vi "PB_Nest_Loops.vi"(2 "error in (no error)":errorcluster, 3 "PB VLIW Array in":T1(array[cluster]) {"Output Bits" format="%x"}) -> (0 "error out":errorcluster, 1 "PB VLIW Array out":T1(array[cluster]) {"Output Bits" format="%x"})   [LabVIEW 2013, in "PulseBlaster.lvlib"]
uses:
  PulseBlaster.lvlib
  <vilib>/ErrorRing/Error Ring.xnode
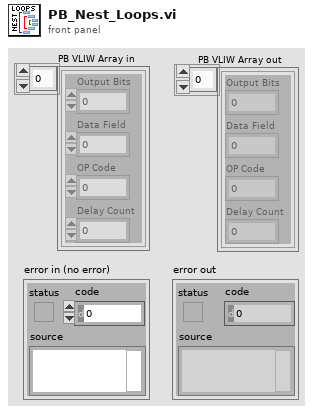
[diagram p1: front panel]
types:
  T1 = cluster{"Output Bits":u32, "Data Field":u32, "OP Code":u8, "Delay Count":u64}[]
  T2 = cluster{"Output Bits":u32, "Data Field":u32, "OP Code":u8, "Delay Count":u64}
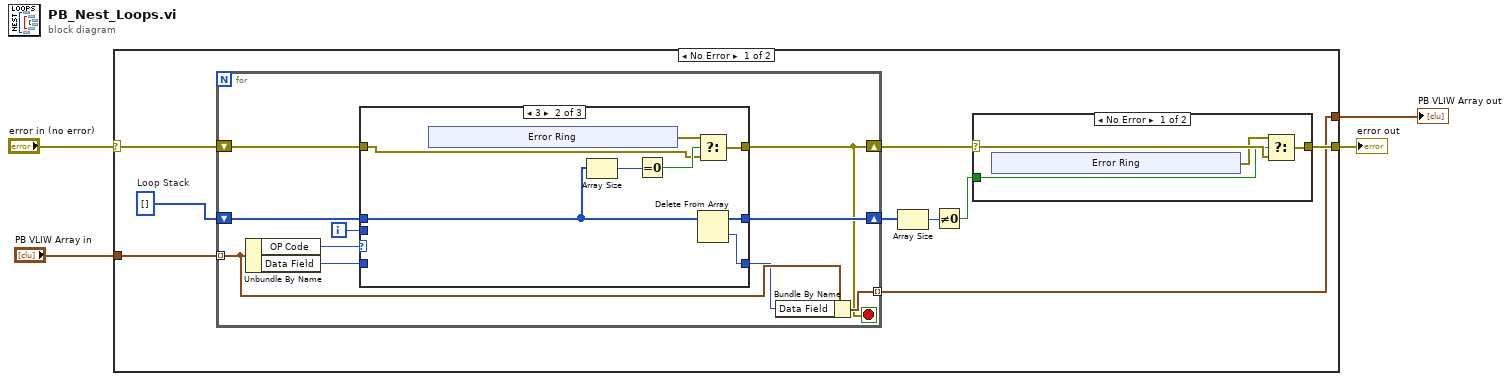
[diagram p0: block diagram]
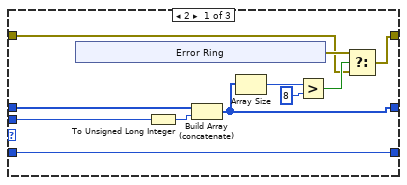
[diagram p3: hidden frame]
diagram:
  n1 = case shown="No Error" "error in (no error)" {
    selector: "error in (no error)" -> [w13 w55]
    tunnel: [w9 w55] -> w3
    tunnel: "PB VLIW Array in" -> [w12 w54]
    tunnel: [w5 w54] -> w1
    frame No Error {
      w11 = u32[] []  # Loop Stack
      n2 = for {
        shift-right: [w20] -> w10
        shift-left: w13 -> [w22]
        shift-right: [w23] -> w7
        shift-left: w11 -> [w24]
        tunnel: w12 -> [w28] mode=indexing
        tunnel: [w21] -> w5 mode=indexing
        i -> [w27]
        stop <- w20 stop-if-true
        n3 = Unbundle By Name(w28) -> ("OP Code"=w25:u8, "Data Field"=w29:u32)
        n4 = case shown="3" w25 {
          tunnel: [w40 w45 w52] -> w23
          tunnel: [w35 w46 w51] -> w20
          tunnel: w29 -> [w32 _ w53]
          tunnel: w27 -> [w33 _ _]
          tunnel: [w32 w42 w53] -> w26
          tunnel: w24 -> [w31 w44 w52]
          tunnel: w22 -> [w30 w43 w51]
          frame 2 {
            n5 = xnode "Error Ring"() -> ("error out"=w36:errorcluster)
            n6 = To Unsigned Long Integer(number=w33) -> (unsigned 32bit integer=w34:u32)
            n7 = Build Array (concatenate)(w31, w34) -> (w40:u32[])
            n8 = Array Size(array=w40) -> (size(s)=w39:i32)
            n9 = Greater?(x=w39, y=8) -> (0:w37:bool)
            n10 = Select(t=w36, s=w37, f=w30) -> (s? t:f=w35:errorcluster)
          }
          frame 3 {
            n11 = xnode "Error Ring"() -> ("error out"=w47:errorcluster)
            n12 = Array Size(array=w44) -> (size(s)=w49:i32)
            n13 = Equal To 0?(x=w49) -> (x = 0?=w48:bool)
            n14 = Select(t=w47, s=w48, f=w43) -> (s? t:f=w46:errorcluster)
            n15 = Delete From Array(array=w44) -> (deleted portion=w42:u32, array with subset deleted=w45:u32[])  [unwired: 2 in]
          }
          frame Default {
          }
        }
        n16 = Bundle By Name(cluster=w28, "Data Field"=w26) -> (w21:T2)
      }
      n17 = Array Size(array=w7) -> (size(s)=w6:i32)
      n18 = Not Equal To 0?(x=w6) -> (x != 0?=w8:bool)
      n19 = case shown="No Error" w10 {
        selector: w10 -> [w17 w19]
        tunnel: [w16 w19] -> w9
        tunnel: w8 -> [w14 _]
        frame No Error {
          n20 = xnode "Error Ring"() -> ("error out"=w15:errorcluster)
          n21 = Select(t=w15, s=w14, f=w17) -> (s? t:f=w16:errorcluster)
        }
        frame Error {
        }
      }
    }
    frame Error {
    }
  }
  "error out" <- w3
  "PB VLIW Array out" <- w1
